vi "Digital Input Data.vi"(8 "error in (no error)":errorcluster, 10 "Digital Data":bool[](array[boolean]), 11 "DAQmx Actor Interface in":refnum<class "DAQmx Actor Interface.lvclass">) -> (0 "error out":errorcluster, 3 "DAQmx Actor Interface out":refnum<class "DAQmx Actor Interface.lvclass">)   [LabVIEW 2024, in "DAQmx Actor Interface.lvlib" / "DAQmx Actor Interface.lvclass"]
uses:
  DAQmx Actor Interface.lvclass
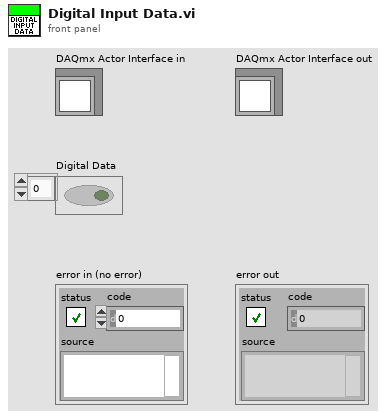
[diagram p1: front panel]
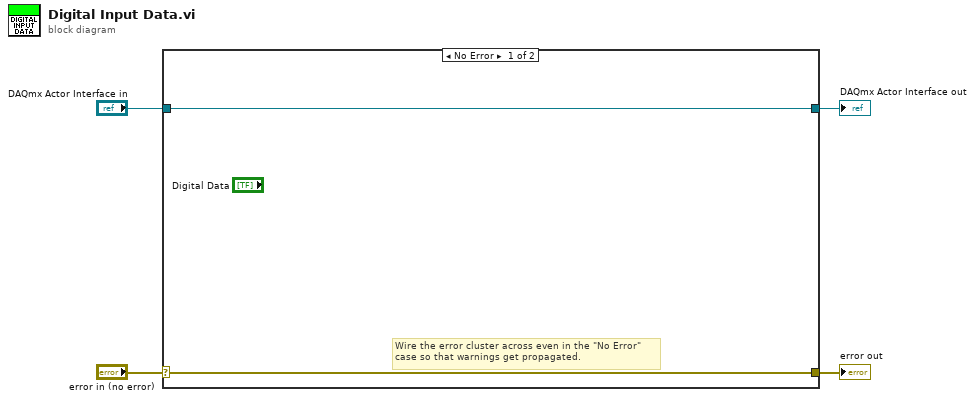
[diagram p0: block diagram]
diagram:
  n1 = case shown="No Error" "error in (no error)" {
    selector: "error in (no error)" -> [w5 w8]
    tunnel: [w5 w8] -> w3
    tunnel: [w6 w7] -> w1
    tunnel: "DAQmx Actor Interface in" -> [w6 w7]
    frame No Error {
      # "Wire the error cluster across even in the \"No Error\"\ncase so that warnings get propagated."
    }
    frame Error {
    }
  }
  "error out" <- w3
  "DAQmx Actor Interface out" <- w1
